vi "8HP_Pressures_to UVW.vi"(0 "Probe Number":i32) -> ()   [LabVIEW 2018]
uses:
  Controls/Setup.ctl
  Globals/Meas_global.vi
panel:
  out "Relative yaw (deg)":sgl
  out "Relative pitch (deg)":sgl
  out "Relative roll (deg)":sgl
  out "Calib. pitch (deg)":sgl
  out "Calib. roll (deg)":sgl
  out "Pitch (deg)":sgl
  out "Roll (deg)":sgl
  in  "Desired Freq Hz":dbl=50.0
  out "Averaging samples":i32=5
  out "Current Case":string
  out "UVW chs":i32[](array[numeric])
  out "UVW":sgl[][](array[numeric])
  out "8 Hole Probe chs":string[](array[string])
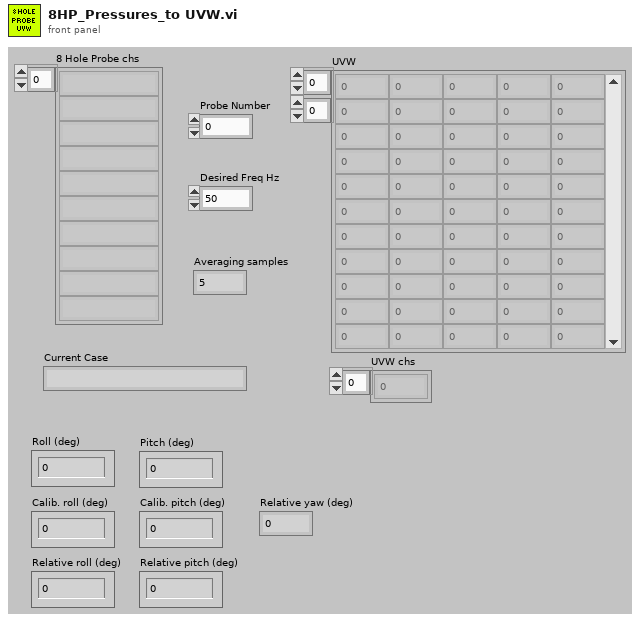
[diagram p1: front panel]
types:
  T1 = typedef "Analysis_info_cluster.ctl" = cluster{"Colour":u32, "Inst type":T2, "Inst name":string, "Symbol":string, "Code name":string, "Extra Info":string, "Inst Array":T3, "Extra Titles":string[], "Extra Values":string[], "U":dbl, "u^2":dbl, "u^3":dbl, "u^4":dbl, "Skew_u":dbl, "Kurt_u":dbl, "Sd Error in Mean":dbl, "% u'/U":dbl, "X":dbl, "Y":dbl, "Z":dbl, "Timescale integral Estimate":dbl, "Sd Error in Variance":dbl, "Calib File":path, "Calib Constants":dbl[], "Output Position":bool, "Stats":enum16{"None", "Basic", "Full"}, "Av Sampling Rate":dbl, "Av No of Samples":dbl, "Total Meas Time (s)":dbl, "ADAM Ch Name":string, "Max value":dbl, "Min value":dbl, "Req Sample Rate Hz":dbl, "Sync Delay Time (s)":dbl, "Ch No":i16, "Device":string, "Use Latest Calib":bool, "Port":string, "Metadata Ch Names":string[], "Metadata Ch Values":string[]}
  T2 = typedef "Inst_type.ctl" = enum16{"Propeller anemometer", "Raw voltage", "Pressure Transducer", "Pitot-static tube", "Preston tube", "Hot wire", "Cross wire 1", "Cross wire 2", "Generic Linear", "Generic Polynomial", "Generic BackPoly", "Fast FID", "Thermocouple", "Cold wire", "Pulsed Wire", "LDA Vel", "LDA Tran time", "LDA Arr time", "Microphone"}
  T3 = typedef "Instrument_Array.ctl" = enum16{"PWA", "LDA", "Analogue"}
  T4 = typedef "Time_Trace_Cluster.ctl" = cluster{"Weighting":dbl[], "Time (s)":dbl[], "Voltage":dbl[], "Eng Values":dbl[]}
  T5 = typedef "Setup.ctl" = enum16{"Run Program", "Show Setup", "Save Current Setup", "Setup Front Panel"}
  T6 = cluster{"Pressure Ch Names":string[], "Pressure Index":i32[], "Metadata Index":i32[], "Port":string}[]
  T7 = cluster{"Pressure Ch Names":string[], "Pressure Index":i32[], "Metadata Index":i32[], "Port":string}
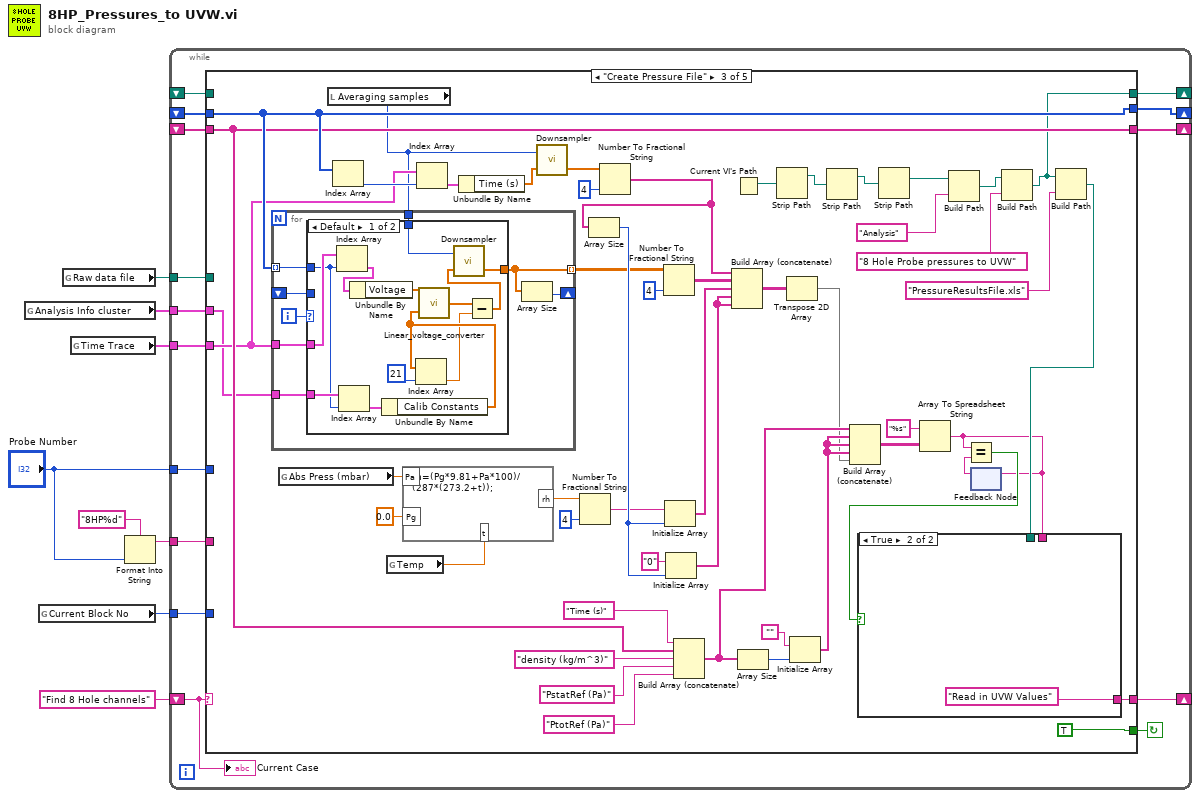
[diagram p0: block diagram]
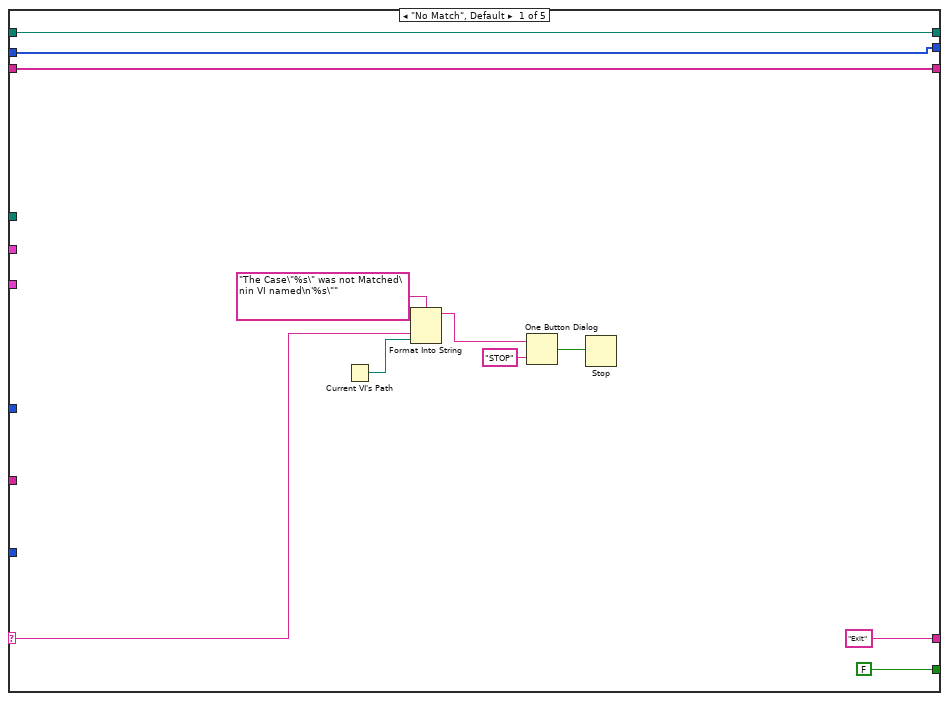
[diagram p2: hidden frame]
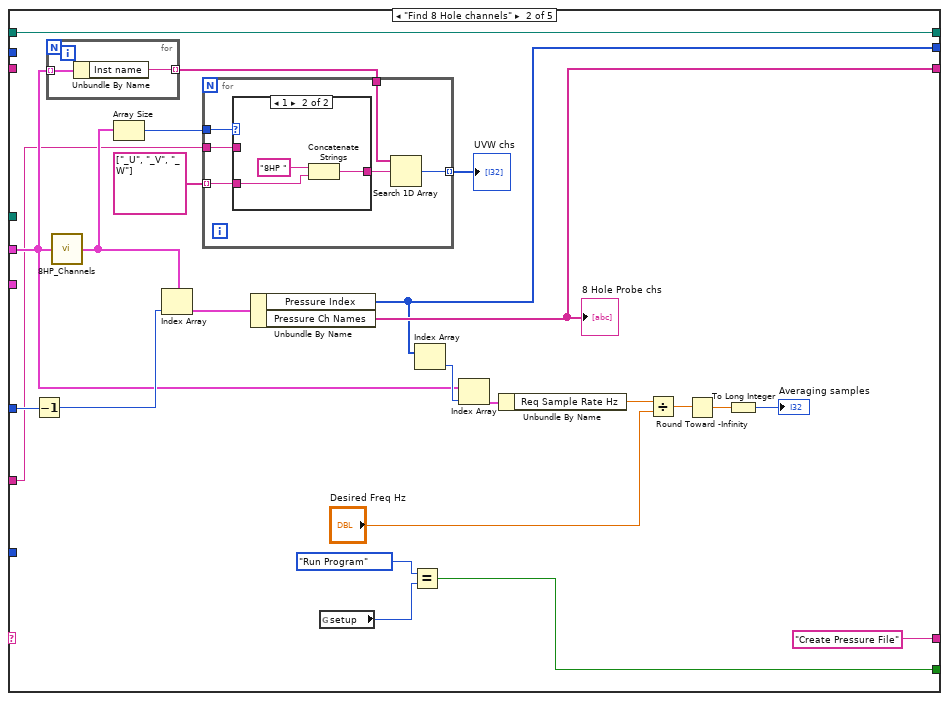
[diagram p3: hidden frame]
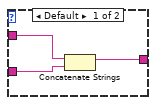
[diagram p4: hidden frame]
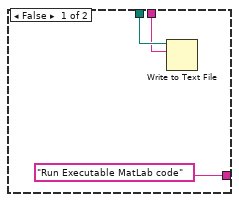
[diagram p5: hidden frame]
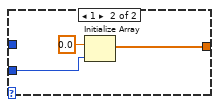
[diagram p6: hidden frame]
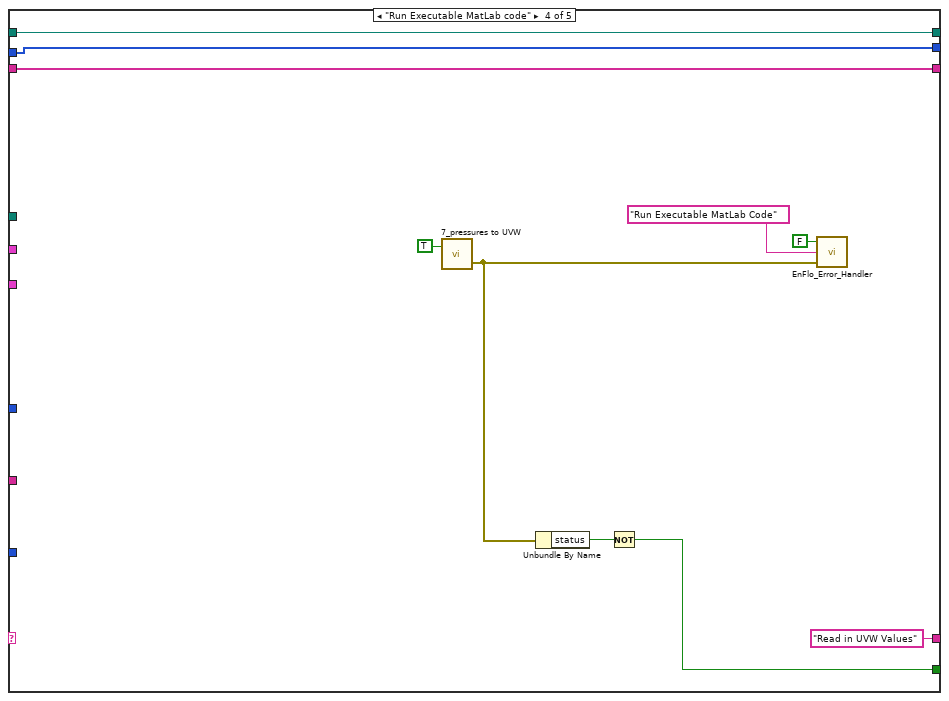
[diagram p7: hidden frame]
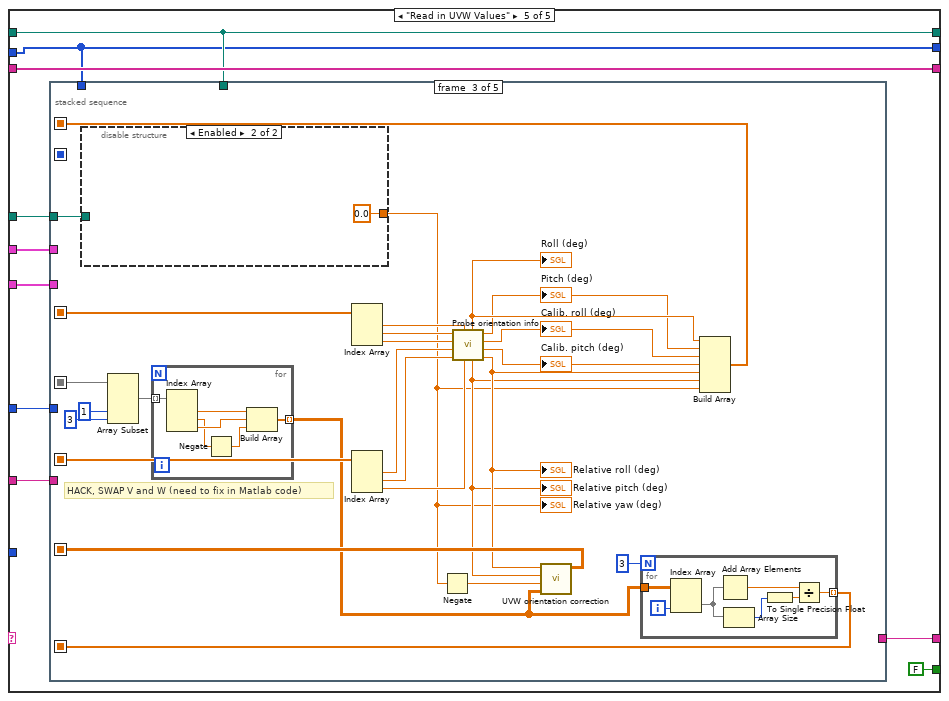
[diagram p8: hidden frame]
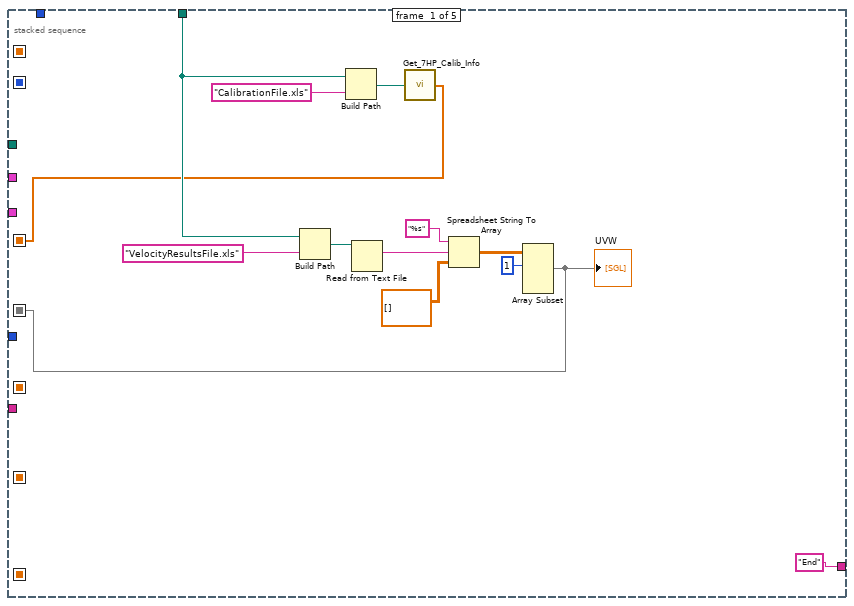
[diagram p9: hidden frame]
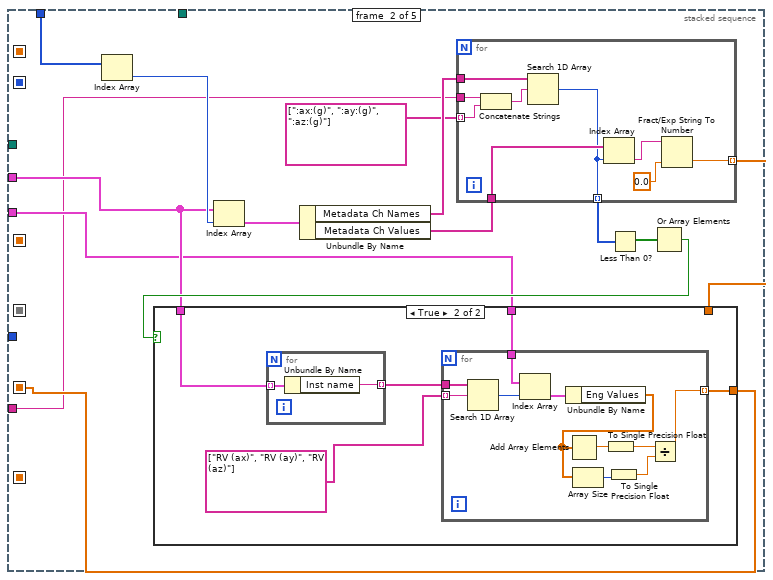
[diagram p10: hidden frame]
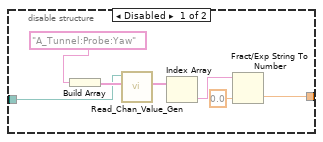
[diagram p12: hidden frame]
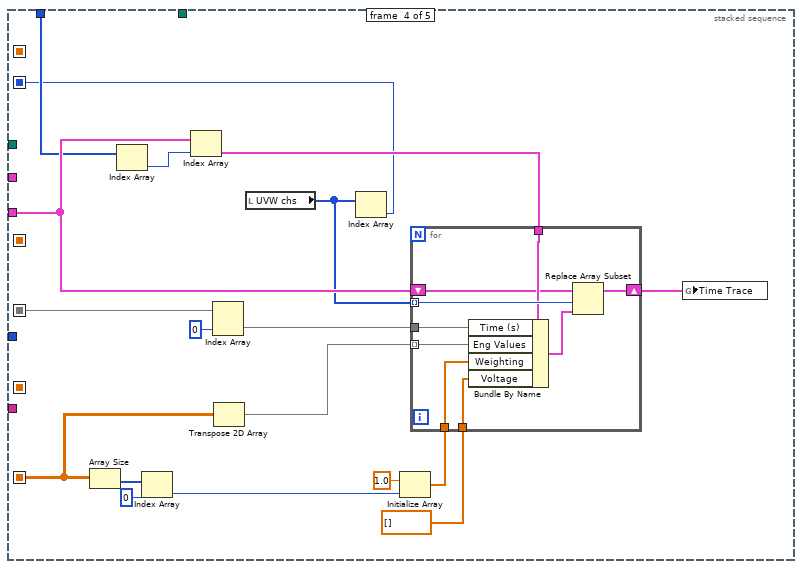
[diagram p13: hidden frame]
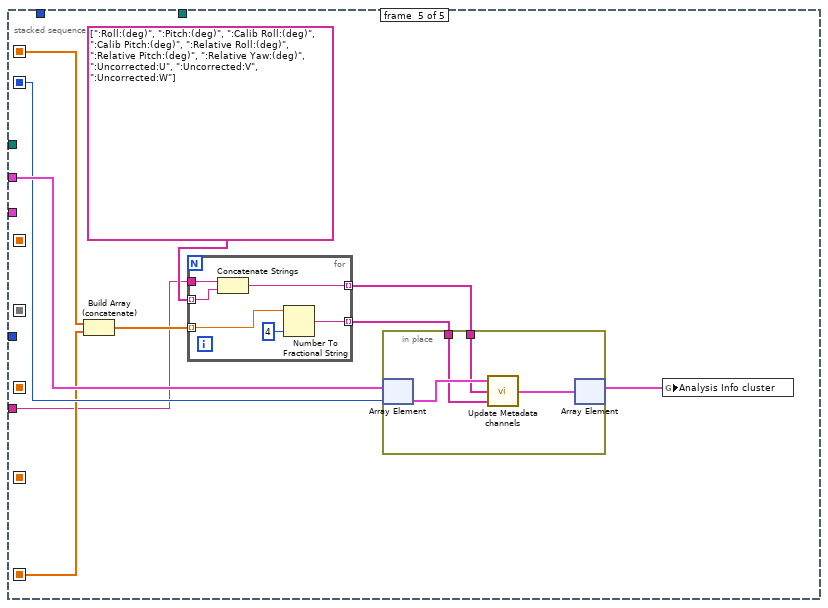
[diagram p14: hidden frame]
diagram:
  n1 = global read "Meas_global.vi" "Analysis Info cluster"() -> (w6:T1[])
  n2 = global read "Meas_global.vi" "Current Block No"() -> (w4:i32)
  n3 = global read "Meas_global.vi" "Raw data file"() -> (w7:path)
  n4 = global read "Meas_global.vi" "Time Trace"() -> (w5:T4[])
  n5 = Format Into String(format string="8HP%d", "Probe Number") -> (resulting string=w2:string)  [unwired: 2 in, 1 out]
  n6 = while {
    shift-left: "Find 8 Hole channels" -> [w11]
    shift-right: [w12] -> _
    tunnel: w7 -> [w22]
    tunnel: w6 -> [w21]
    shift-right: [w20] -> _
    shift-left: _ -> [w19]
    shift-right: [w18] -> _
    shift-left: _ -> [w17]
    shift-right: [w16] -> _
    shift-left: _ -> [w15]
    tunnel: w5 -> [w14]
    tunnel: w4 -> [w13]
    tunnel: "Probe Number" -> [w10]
    tunnel: w2 -> [w9]
    stop <- w23 continue-if-true
    n7 = case shown="\"Create Pressure File\"" w11 {
      selector: w11 -> [w24 _ _ _ _]
      tunnel: [FALSE w54 TRUE w153 FALSE] -> w23
      tunnel: ["Exit" "Create Pressure File" ("t") w122 "Read in UVW Values" ("t") w168] -> w12
      tunnel: w22 -> [_ _ _ _ w164]
      tunnel: w21 -> [_ w39 w73 _ w165]
      tunnel: [w27 w51 w121 w152 w166] -> w20
      tunnel: w19 -> [w27 _ w121 w152 w166]
      tunnel: [w26 w52 w96 w161 w171] -> w18
      tunnel: w17 -> [w26 _ w96 w161 w171]
      tunnel: [w25 w57 w83 w157 w169] -> w16
      tunnel: w15 -> [w25 w57 _ w157 w169]
      tunnel: w14 -> [_ _ w82 _ w167]
      tunnel: w13 -> [_ _ _ _ _]
      tunnel: w10 -> [_ w36 _ _ w163]
      tunnel: w9 -> [_ w35 _ _ w162]
      frame "No Match", Default {
        n8 = Current VI's Path() -> (path=w29:path)
        n9 = Format Into String(format string="The Case\"%s\" was not Matched\nin VI named\n'%s\"" ("Format String"), w24, w29) -> (resulting string=w32:string)  [unwired: 2 in, 1 out]
        n10 = One Button Dialog(message=w32, button name ("OK")="STOP") -> (true=w30:bool)
        n11 = Stop(stop? (T)=w30) -> ()
      }
      frame "Find 8 Hole channels" {
        n12 = Decrement(x=w36) -> (x-1=w43:i32)
        n13 = for {
          tunnel: w39 -> [w60] mode=indexing
          tunnel: [w59] -> w38 mode=indexing
          n14 = Unbundle By Name(w60) -> ("Inst name"=w59:string)
        }
        n15 = call "8HP_Channels.vi"("Analysis Info cluster"=w39) -> ("8HP Info"=w42:T6)
        n16 = Array Size(array=w42) -> (size(s)=w41:i32)
        n17 = Index Array(array=w42, index=w43) -> (element=w53:T7)
        n18 = for {
          tunnel: w41 -> [w66]
          tunnel: string[] ["_U", "_V", "_W"] ("appended array") -> [w65] mode=indexing
          tunnel: w38 -> [w64]
          tunnel: [w62] -> w37 mode=indexing
          tunnel: w35 -> [w61]
          n19 = case shown="1" w66 {
            tunnel: w65 -> [w69 w71]
            tunnel: [w67 w70] -> w63
            tunnel: w61 -> [w68 _]
            frame Default {
              n20 = Concatenate Strings(w68, w69) -> (w67:string)
            }
            frame 1 {
              n21 = Concatenate Strings("8HP " ("Inst name"), w71) -> (w70:string)
            }
          }
          n22 = Search 1D Array(1D array=w64, element=w63) -> (index of element=w62:i32)  [unwired: 1 in]
        }
        "UVW chs" <- w37
        n23 = Unbundle By Name(w53) -> ("Pressure Index"=w51:i32[], "Pressure Ch Names"=w52:string[])
        "8 Hole Probe chs" <- w52
        n24 = global read "Meas_global.vi" "setup"() -> (w56:T5)
        n25 = Equal?(x=Setup."Run Program" ("setup"), y=w56) -> (x = y?=w54:bool)
        n26 = Index Array(array=w51) -> (element=w50:i32)  [unwired: 1 in]
        n27 = Index Array(array=w39, index=w50) -> (element=w49:T1)
        n28 = Unbundle By Name(w49) -> ("Req Sample Rate Hz"=w48:dbl)
        n29 = Divide(x=w48, y="Desired Freq Hz") -> (x/y=w46:dbl)
        n30 = Round Toward -Infinity(1:w46) -> (0:w45:dbl)
        n31 = To Long Integer(number=w45) -> (32bit integer=→"Averaging samples":i32)
      }
      frame "Create Pressure File" {
        n32 = global read "Meas_global.vi" "Abs Press (mbar)"() -> (w117:dbl)
        n33 = local read "Averaging samples"() -> (w76:i32)
        n34 = for {
          tunnel: w121 -> [w135] mode=indexing
          tunnel: [w133] -> w104 mode=indexing
          tunnel: w82 -> [w129]
          tunnel: w76 -> [w134]
          shift-right: [w132] -> _
          shift-left: _ -> [w130]
          tunnel: w73 -> [w128]
          i -> [w131]
          n35 = case shown="Default" w131 {
            tunnel: w135 -> [w143 _]
            tunnel: w134 -> [w147 _]
            tunnel: [w146 w149] -> w133
            tunnel: w130 -> [_ w151]
            tunnel: w129 -> [w145 _]
            tunnel: w128 -> [w144 _]
            frame Default {
              n36 = Index Array(array=w145, index=w143) -> (element=w148:T4)
              n37 = Index Array(array=w144, index=w143) -> (element=w142:T1)
              n38 = Unbundle By Name(w148) -> ("Voltage"=w141:dbl[])
              n39 = Unbundle By Name(w142) -> ("Calib Constants"=w137:dbl[])
              n40 = Index Array(array=w137, index=21) -> (element=w136:dbl)
              n41 = call "Linear_voltage_converter.vi"("Caib const A,B"=w137, "Voltage array"=w141) -> ("Converted array"=w140:dbl[])
              n42 = Subtract(x=w140, y=w136) -> (x-y=w139:dbl[])
              n43 = call "Downsampler.vi"("Input Array"=w139, "Averaging samples"=w147) -> ("Downsampled Array"=w146:dbl[])  [unwired: 1 out]
            }
            frame 1 {
              n44 = Initialize Array(0.0 ("element"), w151) -> (w149:dbl[])
            }
          }
          n45 = Array Size(array=w133) -> (size(s)=w132:i32)
        }
        n46 = Index Array(array=w121) -> (element=w119:i32)  [unwired: 1 in]
        n47 = global read "Meas_global.vi" "Temp"() -> (w118:dbl)
        n48 = formula code="rh=(Pg*9.81+Pa*100)/\n(287*(273.2+t));"("t"=w118, "Pg"=0.0 ("input variable"), "Pa"=w117) -> ("rh"=w101:dbl)
        n49 = Index Array(array=w82, index=w119) -> (element=w120:T4)
        n50 = Unbundle By Name(w120) -> ("Time (s)"=w78:dbl[])
        n51 = call "Downsampler.vi"("Input Array"=w78, "Averaging samples"=w76) -> ("Downsampled Array"=w77:dbl[])  [unwired: 1 out]
        n52 = Number To Fractional String(number=w101, precision (6)=i16 4) -> (F-format string=w100:string)  [unwired: 2 in]
        n53 = Number To Fractional String(number=w77, precision (6)=i16 4) -> (F-format string=w106:string[])  [unwired: 2 in]
        n54 = Array Size(array=w106) -> (size(s)=w115:i32)
        n55 = Number To Fractional String(number=w104, precision (6)=i16 4) -> (F-format string=w103:string[][])  [unwired: 2 in]
        n56 = Initialize Array(w100, w115) -> (w113:string[])
        n57 = Initialize Array("0" ("element"), w115) -> (w112:string[])
        n58 = Build Array (concatenate)("Time (s)", w96, "density (kg/m^3)", "PstatRef (Pa)", "PtotRef (Pa)") -> (w88:string[])
        n59 = Build Array (concatenate)(w106, w103, w113, w112, w112) -> (w99:string[][])
        n60 = Current VI's Path() -> (path=w95:path)
        n61 = Array Size(array=w88) -> (size(s)=w87:i32)
        n62 = Strip Path(path=w95) -> (stripped path=w94:path)  [unwired: 1 out]
        n63 = Transpose 2D Array(2D array=w99) -> (transposed array=w84:string[][])
        n64 = Initialize Array("", w87) -> (w85:string[])
        n65 = Strip Path(path=w94) -> (stripped path=w75:path)  [unwired: 1 out]
        n66 = Build Array (concatenate)(w88, w85, w85, w85, w84) -> (w98:string[][])
        n67 = Strip Path(path=w75) -> (stripped path=w74:path)  [unwired: 1 out]
        n68 = Array To Spreadsheet String(array=w98, 3:"%s" ("format string")) -> (spreadsheet string=w79:string)  [unwired: 1 in]
        n69 = Build Path(base path=w74, name or relative path="Analysis") -> (appended path=w92:path)
        n70 = feedback-in #1(w79) -> ()
        n71 = feedback #1() -> (w81:string)  [unwired: 1 in]
        n72 = Equal?(x=w79, y=w81) -> (x = y?=w80:bool)
        n73 = Build Path(base path=w92, name or relative path="8 Hole Probe pressures to UVW") -> (appended path=w83:path)
        n74 = Build Path(base path=w83, name or relative path="PressureResultsFile.xls") -> (appended path=w89:path)
        n75 = case shown="True" w80 {
          tunnel: ["Run Executable MatLab code" ("t") "Read in UVW Values" ("t")] -> w122
          tunnel: w89 -> [w126 _]
          tunnel: w79 -> [w125 _]
          frame False {
            n76 = Write to Text File(file (use dialog)=w126, text=w125) -> ()  [unwired: 2 in, 3 out]
          }
          frame True {
          }
        }
      }
      frame "Run Executable MatLab code" {
        n77 = call "7_pressures to UVW.vi"("wait until completion?"=TRUE) -> ("error out"=w155:errorcluster)  [unwired: 2 in]
        n78 = Unbundle By Name(w155) -> ("status"=w154:bool)
        n79 = Not(x=w154) -> (.not. x?=w153:bool)
        n80 = call "EnFlo_Error_Handler.vi"("error in (no error)"=w155, "Error Type"="Run Executable MatLab Code", "Dialog Box (T)"=FALSE) -> ()  [unwired: 3 out]
      }
      frame "Read in UVW Values" {
        n81 = stacked-sequence {
          seq-local: [w176 _ _ _ _] -> [_ _ w247 w281 _]
          seq-local: [_ w188 _ _ _] -> [_ _ w252 _ _]
          seq-local: [_ _ w248 _ _] -> [_ _ _ w275 _]
          seq-local: [_ _ w241 _ _] -> [_ _ _ _ w303]
          seq-local: [_ _ _ w279 _] -> [_ _ _ _ w308]
          seq-local: [_ _ w239 _ _] -> [_ _ _ _ w304]
          seq-local: [w172 _ _ _ _] -> [_ _ w233 _ _]
          tunnel: w169 -> [w174 _ _ _ _]
          tunnel: ["End" ("t") _ _ _ _] -> w168
          tunnel: w167 -> [_ w186 _ w283 _]
          tunnel: w166 -> [_ w198 _ w282 _]
          tunnel: w165 -> [_ w189 _ _ w309]
          tunnel: w164 -> [_ _ w238 _ _]
          tunnel: w163 -> [_ _ _ _ _]
          tunnel: w162 -> [_ w185 _ _ w301]
          frame #0 {
            n82 = Build Path(base path=w174, name or relative path="VelocityResultsFile.xls") -> (appended path=w183:path)
            n83 = Build Path(base path=w174, name or relative path="CalibrationFile.xls") -> (appended path=w173:path)
            n84 = Read from Text File(file (use dialog)=w183) -> (text=w182:string)  [unwired: 3 in, 3 out]
            n85 = call "Get_7HP_Calib_Info.vi"("Results file"=w173) -> ("ax ay az"=w172:sgl[])
            n86 = Spreadsheet String To Array(format string="%s", spreadsheet string=w182, array type (2D Dbl)=sgl[][] []) -> (array=w179:sgl[][])  [unwired: 1 in]
            n87 = Array Subset(array=w179, index (row)=1 ("index")) -> (w176:sgl[][])  [unwired: 3 in]
            "UVW" <- w176
          }
          frame #1 {
            n88 = Index Array(array=w198) -> (element=w197:i32)  [unwired: 1 in]
            n89 = Index Array(array=w189, index=w197) -> (element=w196:T1)
            n90 = Unbundle By Name(w196) -> ("Metadata Ch Names"=w195:string[], "Metadata Ch Values"=w193:string[])
            n91 = for {
              tunnel: w195 -> [w226]
              tunnel: string[] [":ax:(g)", ":ay:(g)", ":az:(g)"] ("Metadata Ch Names") -> [w220] mode=indexing
              tunnel: w193 -> [w225]
              tunnel: [w223] -> w187 mode=indexing
              tunnel: [w221] -> w192 mode=indexing
              tunnel: w185 -> [w219]
              n92 = Concatenate Strings(w219, w220) -> (w218:string)
              n93 = Search 1D Array(1D array=w226, element=w218) -> (index of element=w221:i32)  [unwired: 1 in]
              n94 = Index Array(array=w225, index=w221) -> (element=w224:string)
              n95 = Fract/Exp String To Number(string=w224, default (0 dbl)=sgl 0.0 ("default (0 DBL)")) -> (number=w223:sgl)  [unwired: 2 in, 1 out]
            }
            n96 = Less Than 0?(x=w192) -> (x < 0?=w191:bool[])
            n97 = Or Array Elements(Boolean array=w191) -> (logical OR=w190:bool)
            n98 = case shown="True" w190 {
              tunnel: w189 -> [_ w202]
              tunnel: [w199 w201] -> w188
              tunnel: w187 -> [w199 _]
              tunnel: w186 -> [_ w200]
              frame False {
              }
              frame True {
                n99 = for {
                  tunnel: w202 -> [w217] mode=indexing
                  tunnel: [w216] -> w204 mode=indexing
                  n100 = Unbundle By Name(w217) -> ("Inst name"=w216:string)
                }
                n101 = for {
                  tunnel: w204 -> [w215]
                  tunnel: string[] ["RV (ax)", "RV (ay)", "RV (az)"] ("Metadata Ch Names") -> [w214] mode=indexing
                  tunnel: w200 -> [w212]
                  tunnel: [w208] -> w201 mode=indexing
                  n102 = Search 1D Array(1D array=w215, element=w214) -> (index of element=w213:i32)  [unwired: 1 in]
                  n103 = Index Array(array=w212, index=w213) -> (element=w211:T4)
                  n104 = Unbundle By Name(w211) -> ("Eng Values"=w209:dbl[])
                  n105 = Add Array Elements(numeric array=w209) -> (sum=w206:dbl)
                  n106 = Array Size(array=w209) -> (size(s)=w207:i32)
                  n107 = To Single Precision Float(number=w206) -> (single precision float=w205:sgl)
                  n108 = To Single Precision Float(number=w207) -> (single precision float=w210:sgl)
                  n109 = Divide(x=w205, y=w210) -> (x/y=w208:sgl)
                }
              }
            }
          }
          frame #2 {
            # "HACK, SWAP V and W (need to fix in Matlab code)"
            n110 = disable-structure shown="Enabled" {
              disable-tunnel: w238 -> [w257 _]
              disable-tunnel: [w253 sgl 0.0 ("Relative yaw (deg)")] -> w227
              frame Disabled {
                n111 = Build Array("A_Tunnel:Probe:Yaw") -> (w258:string[])
                n112 = call "Read_Chan_Value_Gen.vi"("Desired Ch Names"=w258, "Raw data file"=w257) -> ("Values"=w256:string[])  [unwired: 9 in]
                n113 = Index Array(array=w256) -> (element=w255:string)  [unwired: 1 in]
                n114 = Fract/Exp String To Number(string=w255, default (0 dbl)=sgl 0.0 ("default (0 DBL)")) -> (number=w253:sgl)  [unwired: 2 in, 1 out]
              }
              frame Enabled {
              }
            }
            "Relative yaw (deg)" <- w227
            n115 = Array Subset(array=w247, index (col)=1 ("index"), length (col)=3 ("length")) -> (w236:sgl[][])  [unwired: 2 in]
            n116 = for {
              tunnel: w236 -> [w266] mode=indexing
              tunnel: [w264] -> w235 mode=indexing
              n117 = Index Array(array=w266) -> (element #1=w265:sgl, element #2=w262:sgl, element #3=w263:sgl)  [unwired: 3 in]
              n118 = Negate(x=w262) -> (-x=w261:sgl)
              n119 = Build Array(w265, w263, w261) -> (w264:sgl[])
            }
            n120 = Index Array(array=w233) -> (element #1=w232:sgl, element #2=w231:sgl, element #3=w230:sgl)  [unwired: 3 in]
            n121 = Index Array(array=w252) -> (element #1=w251:sgl, element #2=w250:sgl, element #3=w249:sgl)  [unwired: 3 in]
            n122 = Negate(x=w227) -> (-x=w234:sgl)
            n123 = call "Probe orientation info.vi"("az"=w249, "ax_cal"=w232, "ay"=w250, "ax"=w251, "az_cal"=w230, "ay_cal"=w231) -> ("Relative roll (deg)"=w229:sgl, "Calib. pitch (deg)"=w242:sgl, "Calib. roll (deg)"=w237:sgl, "Pitch (deg)"=w243:sgl, "Relative pitch (deg)"=w228:sgl, "Roll (deg)"=w244:sgl)
            "Roll (deg)" <- w244
            "Pitch (deg)" <- w243
            "Calib. roll (deg)" <- w237
            "Calib. pitch (deg)" <- w242
            "Relative roll (deg)" <- w229
            "Relative pitch (deg)" <- w228
            n124 = call "UVW orientation correction.vi"("(U, V, W) array in"=w235, "Relative yaw (deg)"=w234, "Relative pitch (deg)"=w228, "Relative roll (deg)"=w229) -> ("(U, V, W) array out"=w248:sgl[][])  [unwired: 5 in]
            n125 = for {
              N: 3 -> [_]
              tunnel: w235 -> [w273]
              tunnel: [w268] -> w239 mode=indexing
              i -> [w272]
              n126 = Index Array(array=w273, index (col)=w272) -> (element=w271:sgl[])  [unwired: 1 in]
              n127 = Add Array Elements(numeric array=w271) -> (sum=w270:sgl)
              n128 = Array Size(array=w271) -> (size(s)=w269:i32)
              n129 = To Single Precision Float(number=w269) -> (single precision float=w267:sgl)
              n130 = Divide(x=w270, y=w267) -> (x/y=w268:sgl)
            }
            n131 = Build Array(w244, w243, w237, w242, w229, w228, w227) -> (w241:sgl[])
          }
          frame #3 {
            n132 = Array Size(array=w275) -> (size(s)=w278:i32[])
            n133 = Index Array(array=w282) -> (element=w290:i32)  [unwired: 1 in]
            n134 = Index Array(array=w278, index=0) -> (element=w276:i32)
            n135 = Index Array(array=w283, index=w290) -> (element=w289:T4)
            n136 = Index Array(array=w281, index (col)=0 ("disabled index (col)")) -> (element=w288:sgl[])  [unwired: 1 in]
            n137 = Transpose 2D Array(2D array=w275) -> (transposed array=w274:sgl[][])
            n138 = local read "UVW chs"() -> (w280:i32[])
            n139 = Index Array(array=w280) -> (element=w279:i32)  [unwired: 1 in]
            n140 = Initialize Array(1.0 ("element"), w276) -> (w287:dbl[])
            n141 = for {
              tunnel: w280 -> [w300] mode=indexing
              shift-right: [w299] -> w291
              shift-left: w283 -> [w295]
              tunnel: w274 -> [w298] mode=indexing
              tunnel: w289 -> [w296]
              tunnel: w288 -> [w294]
              tunnel: w287 -> [w293]
              tunnel: dbl[] [] ("Voltage") -> [w292]
              n142 = Bundle By Name(cluster=w296, "Time (s)"=w294, "Eng Values"=w298, "Weighting"=w293, "Voltage"=w292) -> (w297:T4)
              n143 = Replace Array Subset(array=w295, new element=w297, index=w300) -> (w299:T4[])
            }
            n144 = global write "Meas_global.vi" "Time Trace"(w291) -> ()
          }
          frame #4 {
            n145 = Build Array (concatenate)(w303, w304) -> (w302:sgl[])
            n146 = for {
              tunnel: w301 -> [w320]
              tunnel: string[] [":Roll:(deg)", ":Pitch:(deg)", ":Calib Roll:(deg)", ":Calib Pitch:(deg)", ":Relative Roll:(deg)", ":Relative Pitch:(deg)", ":Relative Yaw:(deg)", ":Uncorrected:U", ":Uncorrected:V", ":Uncorrected:W"] -> [w319] mode=indexing
              tunnel: w302 -> [w317] mode=indexing
              tunnel: [w316] -> w306 mode=indexing
              tunnel: [w315] -> w305 mode=indexing
              n147 = Concatenate Strings(w320, w319) -> (w316:string)
              n148 = Number To Fractional String(number=w317, precision (6)=i16 4) -> (F-format string=w315:string)  [unwired: 2 in]
            }
            n149 = in-place {
              in-place-border: w306 -> [w312]
              in-place-border: w305 -> [w311]
              n150 = in-place-array #2(w309, w308) -> (w314:T1)
              n151 = call "Update Metadata channels.vi"("Metadata Values"=w311, "Metadata Names"=w312, "Analysis info Cluster in"=w314) -> ("Analysis info Cluster out"=w313:T1)
              n152 = in-place-array #2(w313) -> (w307:T1[])  [unwired: 1 out]
            }
            n153 = global write "Meas_global.vi" "Analysis Info cluster"(w307) -> ()
          }
        }
      }
    }
    "Current Case" <- w11
  }
